vi "Release Queue.vi"(8 "error in (no error)":errorcluster, 11 "ParameterConf in":refnum<class "ParameterConf.lvclass">) -> (0 "error out":errorcluster, 3 "ParameterConf out":refnum<class "ParameterConf.lvclass">)   [LabVIEW 2017, in "LibraryGcode.lvlib" / "ParameterConf.lvclass"]
uses:
  ParameterConf.lvclass
  ParameterConf.lvclass/ParameterConf.ctl
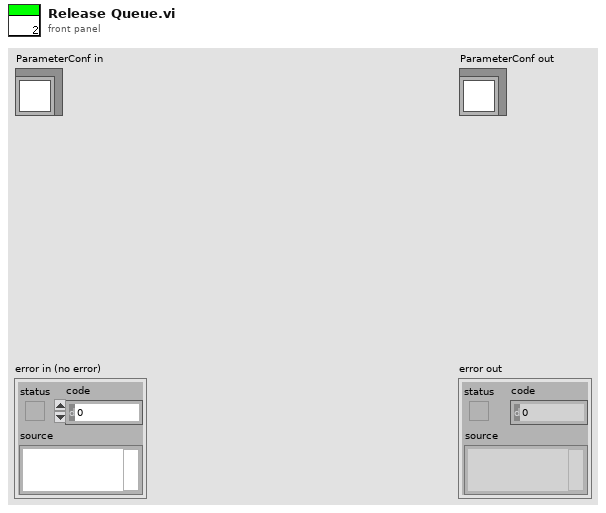
[diagram p1: front panel]
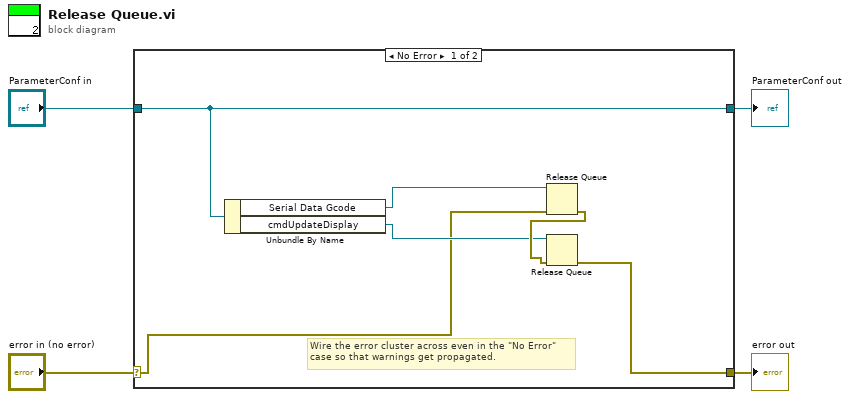
[diagram p0: block diagram]
diagram:
  n1 = case shown="No Error" "error in (no error)" {
    selector: "error in (no error)" -> [w6 w12]
    tunnel: [w7 w12] -> w3
    tunnel: [w5 w11] -> w1
    tunnel: "ParameterConf in" -> [w5 w11]
    frame No Error {
      # "Wire the error cluster across even in the \"No Error\"\ncase so that warnings get propagated."
      n2 = Unbundle By Name(w5) -> ("Serial Data Gcode"=w8:refnum<queue>, "cmdUpdateDisplay"=w9:refnum<queue>)
      n3 = Release Queue(queue=w8, error in (no error)=w6) -> (error out=w10:errorcluster)  [unwired: 1 in, 2 out]
      n4 = Release Queue(queue=w9, error in (no error)=w10) -> (error out=w7:errorcluster)  [unwired: 1 in, 2 out]
    }
    frame Error {
    }
  }
  "error out" <- w3
  "ParameterConf out" <- w1
